vi "Connect.vi"(6 "deadline":T1={"mode"=enum."Relative", "deadline (ms)"=30000}, 8 "error in":errorcluster, 11 "session in":refnum<class "Session.lvclass">) -> (0 "error out":errorcluster, 3 "session out":refnum<class "Session.lvclass">)   [LabVIEW 2020, in "NI_SFTP.lvlib" / "Session.lvclass"]
doc: "Connect to a remote SFTP server. Set the <b>user@host</b> and <b>SSH Client</b> properties before calling this function."
uses:
  <vilib>/net/SFTP/Session/Session.lvclass
  <vilib>/Utility/Deadline/Deadline.ctl
  <vilib>/Utility/Deadline/Mode.ctl
  <vilib>/net/SFTP/Low Level Connection/Low Level Connection.lvclass
  <vilib>/net/SFTP/Session/Session.lvclass/Session.ctl
  <vilib>/net/SSH/Client/Generic/Generic Client.lvclass/Generic Client.ctl
  <vilib>/net/SFTP/Session/Read SSH Client.vi
  <vilib>/net/SFTP/Session/Read user_host.vi
  <vilib>/net/SFTP/Session/Write SSH Client.vi
  <vilib>/net/SSH/Client/Generic/Read trust on first use.vi
  <vilib>/net/SSH/Client/Generic/Generic Client.lvclass
  <vilib>/Utility/Deadline/NI_Deadline.lvlib
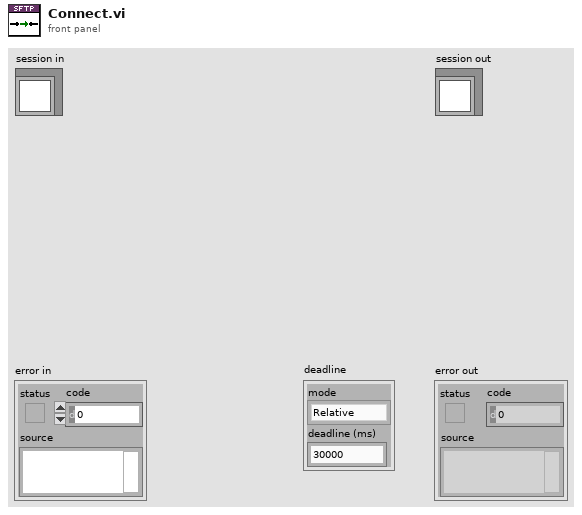
[diagram p1: front panel]
types:
  T1 = typedef "NI_Deadline.lvlib/Deadline.ctl" = cluster{"mode":T2, "deadline (ms)":u32}
  T2 = typedef "NI_Deadline.lvlib/Mode.ctl" = enum16{"Relative", "Use deadline", "Wait forever", "Nonblocking", "N/A"}
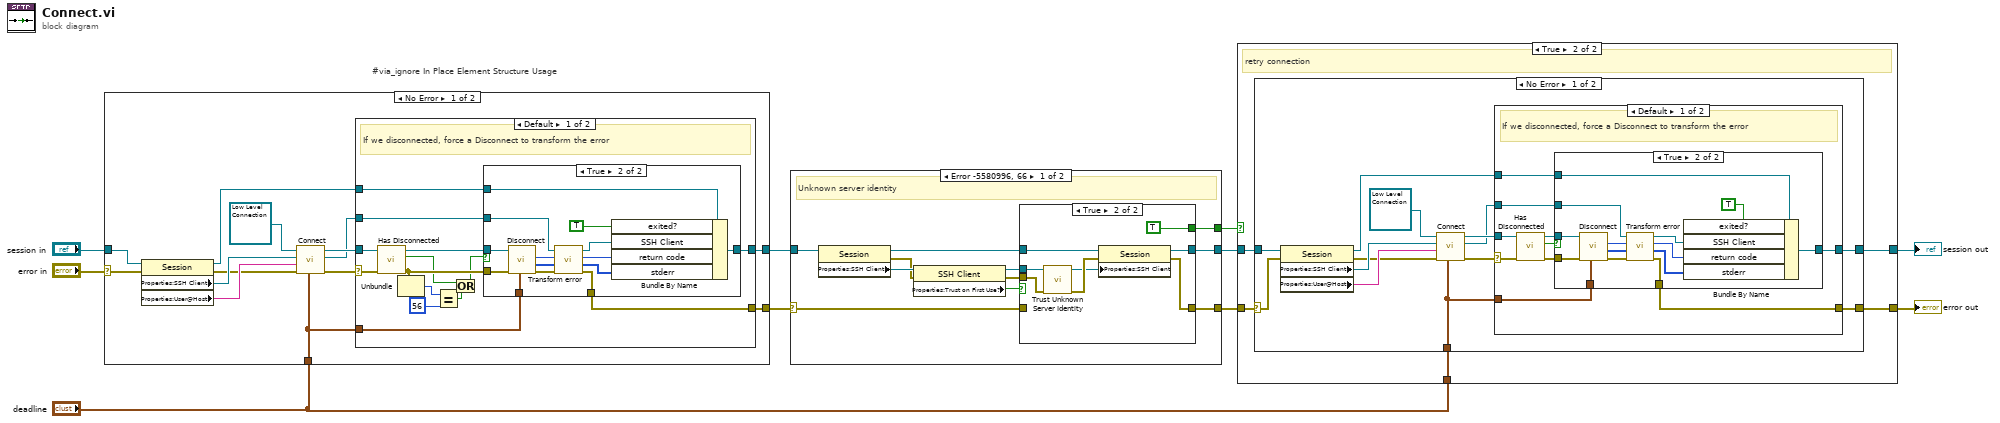
[diagram p0: block diagram]
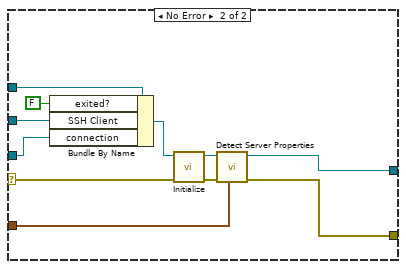
[diagram p6: hidden frame]
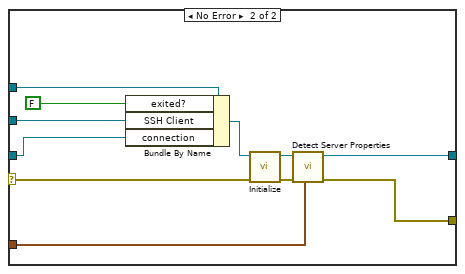
[diagram p9: hidden frame]
diagram:
  # "#via_ignore In Place Element Structure Usage"
  n1 = case shown="No Error" "error in" {
    selector: "error in" -> [w20 w66]
    tunnel: [w11 w66] -> w8
    tunnel: [w13 w65] -> w7
    tunnel: "session in" -> [w23 w65]
    tunnel: "deadline" -> [w12 _]
    frame No Error {
      n2 = property class="Session"(reference=w23, error in=w20) -> (reference out=w14:refnum<class "Session.lvclass">, error out=w19:errorcluster, "Properties:SSH Client"=w22:refnum<class "Generic Client.lvclass">, "Properties:User@Host"=w21:string)
      n3 = call <vilib>:"Connect.vi"("deadline"=w12, "error in"=w19, "user@host"=w21, "client in"=w22, "connection in"=refnum<class "Low Level Connection.lvclass"> refnum ("connection")) -> ("error out"=w17:errorcluster, "session out"=w15:refnum<class "Generic Client.lvclass">, "connection out"=w16:refnum<class "Low Level Connection.lvclass">)  [unwired: 4 in]
      n4 = case shown="Default" w17 {
        selector: w17 -> [w31 w57]
        tunnel: [w30 w56] -> w11
        tunnel: w16 -> [w37 w61]
        tunnel: w15 -> [w35 w62]
        tunnel: w14 -> [w34 w63]
        tunnel: [w33 w55] -> w13
        tunnel: w12 -> [w32 w54]
        frame Default {
          # "If we disconnected, force a Disconnect to transform the error"
          n5 = call <vilib>:"Has Disconnected.vi"("error in (no error)"=w31, "Low Level Connection in"=w37) -> ("error out"=w29:errorcluster, "has disconnected?"=w26:bool, "Low Level Connection out"=w36:refnum<class "Low Level Connection.lvclass">)  [unwired: 7 in]
          n6 = Unbundle(w29) -> ("code"=w28:i32)  [unwired: 2 out]
          n7 = Equal?(x=w28, y=56) -> (x = y?=w25:bool)
          n8 = Or(x=w26, y=w25) -> (x .or. y?=w24:bool)
          n9 = case shown="True" w24 {
            tunnel: w36 -> [_ w53]
            tunnel: w29 -> [w38 w52]
            tunnel: w35 -> [_ w51]
            tunnel: [w38 w47] -> w30
            tunnel: w34 -> [w39 w45]
            tunnel: [w39 w42] -> w33
            tunnel: w32 -> [_ w40]
            frame False {
            }
            frame True {
              n10 = call-dynamic "Disconnect.vi"("deadline"=w40, "error in"=w52, "connection in"=w53) -> ("error out"=w48:errorcluster, "server errors remaining"=w49:u8[], "return code"=w50:u8)  [unwired: 3 in, 3 out]
              n11 = call-dynamic "Transform error.vi"("error in (no error)"=w48, "server errors"=w49, "return code"=w50, "client in"=w51) -> ("error out"=w47:errorcluster, "server errors out"=w41:u8[], "return code out"=w43:u8, "client out"=w44:refnum<class "Generic Client.lvclass">)  [unwired: 4 in]
              n12 = Bundle By Name(cluster=w45, "exited?"=TRUE ("exit info.exited?"), "SSH Client"=w44, "return code"=w43, "stderr"=w41) -> (w42:refnum<class "Session.lvclass">)
            }
          }
        }
        frame No Error {
          n13 = Bundle By Name(cluster=w63, "exited?"=FALSE ("exit info.exited?"), "SSH Client"=w62, "connection"=w61) -> (w58:refnum<class "Session.lvclass">)
          n14 = call <vilib>:"Initialize.vi"("error in"=w57, "session in"=w58) -> ("error out"=w60:errorcluster, "session out"=w59:refnum<class "Session.lvclass">)  [unwired: 8 in]
          n15 = call <vilib>:"Detect Server Properties.vi"("deadline"=w54, "error in"=w60, "session in"=w59) -> ("error out"=w56:errorcluster, "session out"=w55:refnum<class "Session.lvclass">)  [unwired: 7 in]
        }
      }
    }
    frame Error {
    }
  }
  n16 = case shown="Error -5580996, 66" w8 {
    selector: w8 -> [w72 w88]
    tunnel: w7 -> [w77 w89]
    tunnel: [w75 w89] -> w1
    tunnel: [w74 w88] -> w2
    tunnel: [w73 _] -> w3
    frame #0 {
      # "Unknown server identity"
      n17 = property class="Session"(reference=w77) -> (reference out=w76:refnum<class "Session.lvclass">, error out=w68:errorcluster, "Properties:SSH Client"=w70:refnum<class "Generic Client.lvclass">)  [unwired: 1 in]
      n18 = property class="SSH Client"(reference=w70, error in=w68) -> (reference out=w69:refnum<class "Generic Client.lvclass">, error out=w67:errorcluster, "Properties:Trust on First Use?"=w71:bool)
      n19 = case shown="True" w71 {
        tunnel: w67 -> [_ w87]
        tunnel: w69 -> [_ w86]
        tunnel: w76 -> [w79 w85]
        tunnel: [w79 w82] -> w75
        tunnel: [w78 w81] -> w74
        tunnel: [_ TRUE] -> w73
        tunnel: w72 -> [w78 _]
        frame False {
        }
        frame True {
          n20 = call <vilib>:"Trust Unknown Server Identity.vi"("error in (no error)"=w87, "client in"=w86) -> ("error out"=w84:errorcluster, "client out"=w83:refnum<class "Generic Client.lvclass">)  [unwired: 7 in, 1 out]
          n21 = property class="Session"(reference=w85, error in=w84, "Properties:SSH Client"=w83) -> (reference out=w82:refnum<class "Session.lvclass">, error out=w81:errorcluster)
        }
      }
    }
    frame #1 {
    }
  }
  n22 = case shown="True" w3 {
    tunnel: [w90 w96] -> w6
    tunnel: [w91 w95] -> w5
    tunnel: "deadline" -> [_ w94]
    tunnel: w2 -> [w90 w93]
    tunnel: w1 -> [w91 w92]
    frame False {
    }
    frame True {
      # "retry connection"
      n23 = case shown="No Error" w93 {
        selector: w93 -> [w107 w148]
        tunnel: [w98 w148] -> w96
        tunnel: [w100 w147] -> w95
        tunnel: w94 -> [w99 _]
        tunnel: w92 -> [w97 w147]
        frame No Error {
          n24 = property class="Session"(reference=w97, error in=w107) -> (reference out=w101:refnum<class "Session.lvclass">, error out=w106:errorcluster, "Properties:SSH Client"=w109:refnum<class "Generic Client.lvclass">, "Properties:User@Host"=w108:string)
          n25 = call <vilib>:"Connect.vi"("deadline"=w99, "error in"=w106, "user@host"=w108, "client in"=w109, "connection in"=refnum<class "Low Level Connection.lvclass"> refnum ("connection")) -> ("error out"=w104:errorcluster, "session out"=w102:refnum<class "Generic Client.lvclass">, "connection out"=w103:refnum<class "Low Level Connection.lvclass">)  [unwired: 4 in]
          n26 = case shown="Default" w104 {
            selector: w104 -> [w111 w139]
            tunnel: [w110 w138] -> w98
            tunnel: w103 -> [w119 w143]
            tunnel: w102 -> [w115 w144]
            tunnel: w101 -> [w114 w145]
            tunnel: [w113 w137] -> w100
            tunnel: w99 -> [w112 w136]
            frame Default {
              # "If we disconnected, force a Disconnect to transform the error"
              n27 = call <vilib>:"Has Disconnected.vi"("error in (no error)"=w111, "Low Level Connection in"=w119) -> ("error out"=w116:errorcluster, "has disconnected?"=w117:bool, "Low Level Connection out"=w118:refnum<class "Low Level Connection.lvclass">)  [unwired: 7 in]
              n28 = case shown="True" w117 {
                tunnel: w118 -> [_ w135]
                tunnel: w116 -> [w120 w134]
                tunnel: w115 -> [_ w133]
                tunnel: [w120 w129] -> w110
                tunnel: w114 -> [w121 w127]
                tunnel: [w121 w124] -> w113
                tunnel: w112 -> [_ w122]
                frame False {
                }
                frame True {
                  n29 = call-dynamic "Disconnect.vi"("deadline"=w122, "error in"=w134, "connection in"=w135) -> ("error out"=w130:errorcluster, "server errors remaining"=w131:u8[], "return code"=w132:u8)  [unwired: 3 in, 3 out]
                  n30 = call-dynamic "Transform error.vi"("error in (no error)"=w130, "server errors"=w131, "return code"=w132, "client in"=w133) -> ("error out"=w129:errorcluster, "server errors out"=w123:u8[], "return code out"=w125:u8, "client out"=w126:refnum<class "Generic Client.lvclass">)  [unwired: 4 in]
                  n31 = Bundle By Name(cluster=w127, "exited?"=TRUE ("exit info.exited?"), "SSH Client"=w126, "return code"=w125, "stderr"=w123) -> (w124:refnum<class "Session.lvclass">)
                }
              }
            }
            frame No Error {
              n32 = Bundle By Name(cluster=w145, "exited?"=FALSE ("exit info.exited?"), "SSH Client"=w144, "connection"=w143) -> (w140:refnum<class "Session.lvclass">)
              n33 = call <vilib>:"Initialize.vi"("error in"=w139, "session in"=w140) -> ("error out"=w142:errorcluster, "session out"=w141:refnum<class "Session.lvclass">)  [unwired: 8 in]
              n34 = call <vilib>:"Detect Server Properties.vi"("deadline"=w136, "error in"=w142, "session in"=w141) -> ("error out"=w138:errorcluster, "session out"=w137:refnum<class "Session.lvclass">)  [unwired: 7 in]
            }
          }
        }
        frame Error {
        }
      }
    }
  }
  "error out" <- w6
  "session out" <- w5
